vi "Add Missing Pin Error.vi"(6 "pin type":T1, 8 "error in":errorcluster, 9 "instrument type id":string, 10 "site":i32, 11 "missing pin or relay names":string[](array[string])) -> (0 "error out":errorcluster)   [LabVIEW 2020, in "Measurement Plugin Session Management V1.lvlib" / "Session Reservation.lvclass"]
uses:
  Session Reservation.lvclass
  Pin Type.ctl
  MeasurementLink Measurement Server/Helpers/Error Strings Global Internal.vi
  Session Reservation.lvclass/Session Reservation.ctl
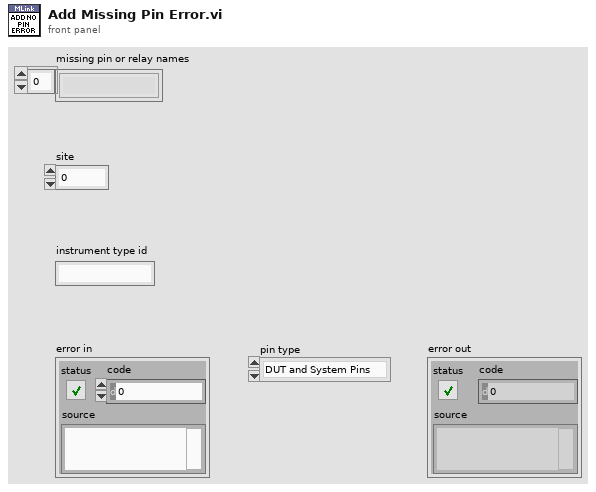
[diagram p1: front panel]
types:
  T1 = typedef "Measurement Plugin Session Management V1.lvlib/Session Reservation.lvclass/Pin Type.ctl" = enum16{"DUT and System Pins", "System Pins"}
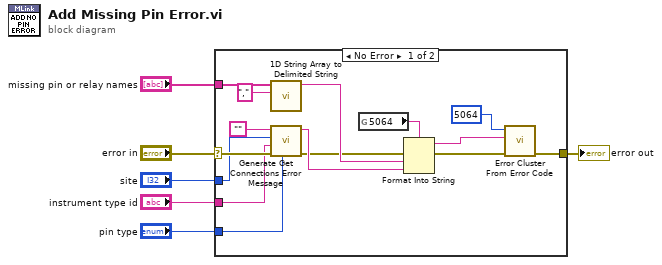
[diagram p0: block diagram]
diagram:
  n1 = case shown="No Error" "error in" {
    selector: "error in" -> [w13 w22]
    tunnel: [w21 w22] -> w5
    tunnel: "missing pin or relay names" -> [w16 _]
    tunnel: "site" -> [w12 _]
    tunnel: "instrument type id" -> [w11 _]
    tunnel: "pin type" -> [w7 _]
    frame No Error {
      n2 = call <vilib>:"1D String Array to Delimited String.vi"("delimiter"=",", "string array"=w16) -> ("delimited string"=w14:string)  [unwired: 9 in]
      n3 = call "Generate Get Connections Error Message.vi"("pin type"=w7, "error in"=w13, "instrument type id"=w11, "site"=w12, "pin or relay names"="") -> ("error out"=w8:errorcluster, "error string"=w9:string)  [unwired: 5 in]
      n4 = global read "Error Strings Global Internal.vi" "5064"() -> (w20:string)
      n5 = Format Into String(format string=w20, error in=w8, w14, w9) -> (resulting string=w17:string, error out=w19:errorcluster)  [unwired: 1 in]
      n6 = call <vilib>:"Error Cluster From Error Code.vi"("error in (no error)"=w19, "error message (\"\")"=w17, "error code (0)"=5064) -> ("error out"=w21:errorcluster)  [unwired: 6 in]
    }
    frame Error {
    }
  }
  "error out" <- w5
